vi "LWConexPSD_Connect.vi"(4 "DiscoverTimeout (10000 msec)":u32=3000, 5 "Launch server? (True)":bool, 6 "Authorize? (True)":bool=TRUE, 7 "Instrument Key":string="CONEX-PSD (A6ULCUPN)") -> (0 "error out":errorcluster, 1 "Instrument Key out":string="CONEX-PSD (A6ULCUPN)", 2 "Component ID":i32=1, 3 "ConexPSD Reference":refnum<k24>)   [LabVIEW 2010]
uses:
  D:/LabVIEW_program/노트북LabVIEW/THz Time/THz Time(SR830_VC_CONEXAGP_nPt_Shot202_2Pt__LGS/Dll/Newport.CONEXPSD.CommandInterface.DLL
  Dll/Newport.CONEXPSD.CommandInterface.DLL
panel:
  in  "error in (no error)":errorcluster
  out "InstrumentKeys":string[](array[string])=["Agilis (FTSK5N2Y)", "CONEX-AGP (A6UFCQ2F)", "CONEX-AGP (A6UFCQ3G)", "CONEX-PSD (A6ULCUPN)", "USB Serial Converter (FTDDH3LZ)"]
  out "ConnectAndDiscover":i32
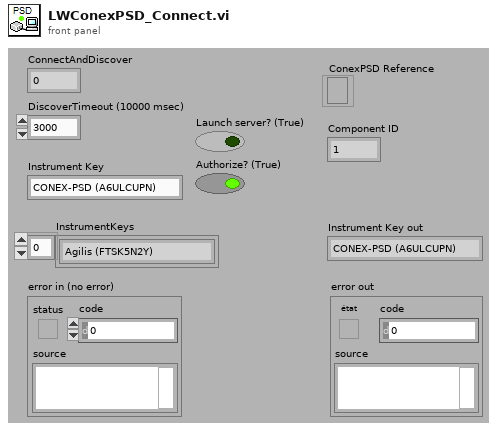
[diagram p1: front panel]
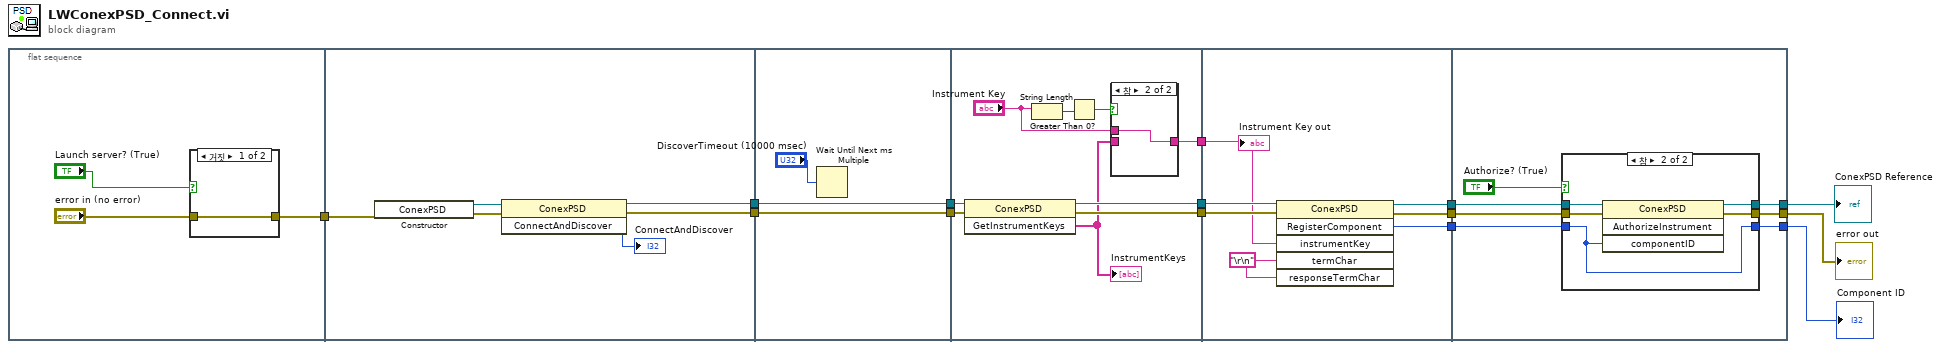
[diagram p0: block diagram]
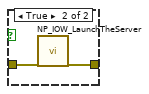
[diagram p2: hidden frame]
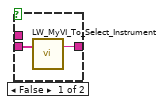
[diagram p3: hidden frame]
diagram:
  n1 = flat-sequence {
    tunnel: [w16] -> w7
    tunnel: [w23] -> w13
    tunnel: [w22] -> w11
    tunnel: w7 -> [w21]
    tunnel: [w28] -> w14
    tunnel: w13 -> [w28]
    tunnel: [w27] -> w12
    tunnel: w11 -> [w27]
    tunnel: w14 -> [w38]
    tunnel: w12 -> [w37]
    tunnel: [w36] -> w6
    tunnel: [w35] -> w5
    tunnel: [w33] -> w4
    tunnel: w6 -> [w48]
    tunnel: w5 -> [w47]
    tunnel: w4 -> [w45]
    tunnel: [w44] -> w3
    tunnel: [w43] -> w2
    tunnel: [w42] -> w1
    tunnel: [w49] -> w8
    tunnel: [w50] -> w9
    tunnel: [w51] -> w10
    tunnel: w3 -> [w54]
    tunnel: w2 -> [w53]
    tunnel: w1 -> [w52]
    frame #0 {
      n2 = case shown="거짓" "Launch server? (True)" {
        tunnel: "error in (no error)" -> [w18 w20]
        tunnel: [w18 w19] -> w16
        frame False {
        }
        frame True {
          n3 = call "NP_IOW_LaunchTheServer.vi"("error in (no error)"=w20) -> ("error out"=w19:errorcluster)  [unwired: 18 in]
        }
      }
    }
    frame #1 {
      n4 = constructor class="ConexPSD"(error in=w21) -> (reference out=w26:refnum<k24>, error out=w25:errorcluster)  [unwired: 2 in, 1 out]
      n5 = invoke class="ConexPSD" method="ConnectAndDiscover"(reference=w26, error in=w25) -> (reference out=w23:refnum<k24>, error out=w22:errorcluster, "ConnectAndDiscover"=→"ConnectAndDiscover":i32)  [unwired: 1 in]
    }
    frame #2 {
      n6 = Wait Until Next ms Multiple(millisecond multiple="DiscoverTimeout (10000 msec)") -> ()  [unwired: 1 out]
    }
    frame #3 {
      n7 = invoke class="ConexPSD" method="GetInstrumentKeys"(reference=w38, error in=w37) -> (reference out=w36:refnum<k24>, error out=w35:errorcluster, "GetInstrumentKeys"=w34:string[])  [unwired: 1 in]
      "InstrumentKeys" <- w34
      n8 = String Length(string="Instrument Key") -> (length=w32:i32)
      n9 = Greater Than 0?(x=w32) -> (x > 0?=w31:bool)
      n10 = case shown="참" w31 {
        tunnel: w34 -> [w40 _]
        tunnel: [w39 w41] -> w33
        tunnel: "Instrument Key" -> [_ w41]
        frame False {
          n11 = call "LW_MyVI_To_Select_Instrument.vi"("Instrument Keys"=w40) -> ("My Instrument Key"=w39:string)  [unwired: 17 in, 1 out]
        }
        frame True {
        }
      }
    }
    frame #4 {
      w46 = "\r\n"
      n12 = invoke class="ConexPSD" method="RegisterComponent"(reference=w48, error in=w47, "instrumentKey"=w45, "termChar"=w46, "responseTermChar"=w46) -> (reference out=w44:refnum<k24>, error out=w43:errorcluster, "RegisterComponent"=w42:i32)  [unwired: 1 in, 3 out]
      "Instrument Key out" <- w45
    }
    frame #5 {
      n13 = case shown="참" "Authorize? (True)" {
        tunnel: w54 -> [w58 w63]
        tunnel: w53 -> [w57 w62]
        tunnel: w52 -> [w56 w59]
        tunnel: [w58 w61] -> w51
        tunnel: [w57 w60] -> w50
        tunnel: [w56 w59] -> w49
        frame False {
        }
        frame True {
          n14 = invoke class="ConexPSD" method="AuthorizeInstrument"(reference=w63, error in=w62, "componentID"=w59) -> (reference out=w61:refnum<k24>, error out=w60:errorcluster)  [unwired: 1 in, 2 out]
        }
      }
    }
  }
  "ConexPSD Reference" <- w10
  "error out" <- w9
  "Component ID" <- w8
